vi "Read Array - String.vi"(8 "error in (no error)":errorcluster, 11 "TAS_Message in":refnum<class "TAS_Message.lvclass">) -> (0 "error out":errorcluster, 2 "Array - String":string[](array[string]), 3 "TAS_Message out":refnum<class "TAS_Message.lvclass">)   [LabVIEW 2012, in "TAS_Message.lvclass"]
uses:
  TAS_Message.lvclass
  TAS_Message.lvclass/TAS_Message.ctl
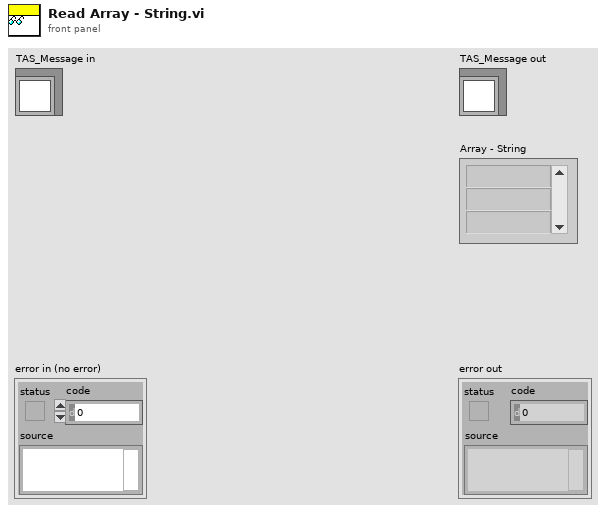
[diagram p1: front panel]
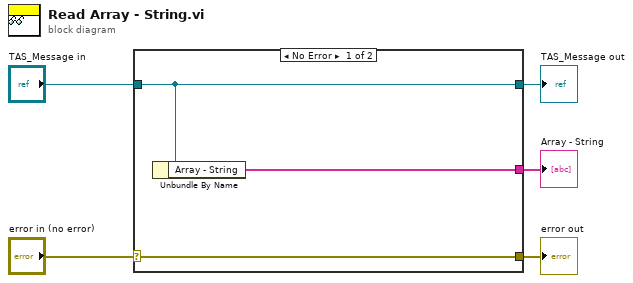
[diagram p0: block diagram]
diagram:
  n1 = case shown="No Error" "error in (no error)" {
    selector: "error in (no error)" -> [w8 w9]
    tunnel: [w8 w9] -> w4
    tunnel: [w7 w10] -> w2
    tunnel: "TAS_Message in" -> [w7 w10]
    tunnel: [w6 _] -> w1
    frame No Error {
      n2 = Unbundle By Name(w7) -> ("Array - String"=w6:string[])
    }
    frame Error {
    }
  }
  "error out" <- w4
  "TAS_Message out" <- w2
  "Array - String" <- w1
